vi "ADCP_UI_Update_Receive_List_Table.vi"(8 "error in (no error)":errorcluster, 11 "ADCU_GUI References":T1) -> ()   [LabVIEW 2017]
uses:
  Controls/ADCP_UI/ADCP_UI_Parameters.ctl
  Controls/ADCP_UI/ADCP_UI_Queues.ctl
  Controls/ADCP_UI/ADCP_UI_Continuous_Receiver_States.ctl
  Controls/ADCP_UI/ADCP_Queue_Receive_Log_Queue_Element.ctl
  Controls/Packet/Packet.ctl
  Controls/Packet/Packet_Direction.ctl
  Controls/Packet/Packet_Type.ctl
  Controls/Packet/Packet_Priority.ctl
  Controls/Data Packets/Data_Packet.ctl
  Controls/Data Packets/Parameter.ctl
  Controls/Data Packets/Parameter_Data_Type.ctl
  Controls/Data Packets/Data_Packet_Transmit_Mode.ctl
  <vilib>/Utility/miscctls.llb/LVRowAndColumnTypeDef.ctl
  ADCP_UI_Receive_List_Data_Packets.vi
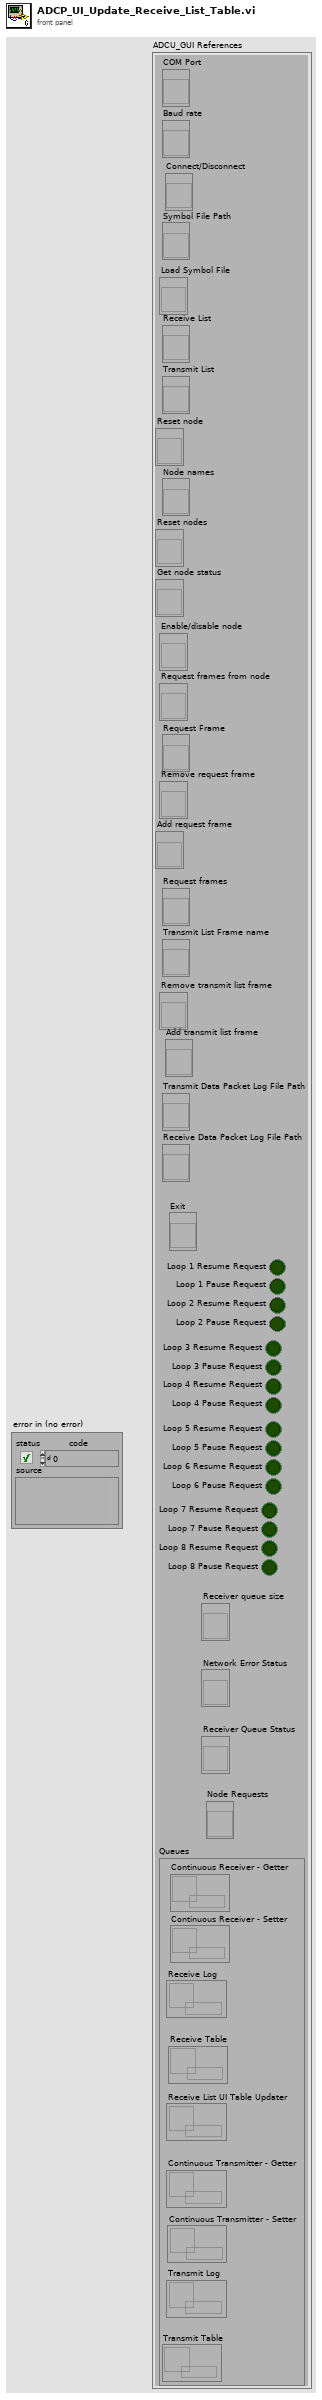
[diagram p1: front panel]
types:
  T1 = typedef "ADCP_UI_Parameters.ctl" = cluster{"COM Port":refnum<vi>, "Baud rate":refnum<vi>, "Symbol File Path":refnum<vi>, "Receive List":refnum<vi>, "Transmit List":refnum<vi>, "Node names":refnum<vi>, "Request Frame":refnum<vi>, "Request frames":refnum<vi>, "Transmit List Frame name":refnum<vi>, "Transmit Data Packet Log File Path":refnum<vi>, "Receive Data Packet Log File Path":refnum<vi>, "Loop 1 Resume Request":bool, "Loop 1 Pause Request":bool, "Loop 2 Resume Request":bool, "Loop 2 Pause Request":bool, "Loop 3 Resume Request":bool, "Loop 3 Pause Request":bool, "Loop 4 Resume Request":bool, "Loop 4 Pause Request":bool, "Loop 5 Resume Request":bool, "Loop 5 Pause Request":bool, "Loop 6 Resume Request":bool, "Loop 6 Pause Request":bool, "Loop 7 Resume Request":bool, "Loop 7 Pause Request":bool, "Loop 8 Resume Request":bool, "Loop 8 Pause Request":bool, "Exit":refnum<vi>, "Connect/Disconnect":refnum<vi>, "Load Symbol File":refnum<vi>, "Reset node":refnum<vi>, "Reset nodes":refnum<vi>, "Get node status":refnum<vi>, "Enable/disable node":refnum<vi>, "Request frames from node":refnum<vi>, "Remove request frame":refnum<vi>, "Add request frame":refnum<vi>, "Remove transmit list frame":refnum<vi>, "Add transmit list frame":refnum<vi>, "Receiver queue size":refnum<vi>, "Network Error Status":refnum<vi>, "Receiver Queue Status":refnum<vi>, "Node Requests":refnum<vi>, "Queues":T2}
  T2 = typedef "ADCP_UI_Queues.ctl" = cluster{"Continuous Receiver - Getter":refnum<queue>, "Continuous Receiver - Setter":refnum<queue>, "Receive Log":refnum<queue>, "Receive Table":refnum<queue>, "Receive List UI Table Updater":refnum<queue>, "Continuous Transmitter - Getter":refnum<queue>, "Continuous Transmitter - Setter":refnum<queue>, "Transmit Log":refnum<queue>, "Transmit Table":refnum<queue>}
  T3 = typedef "Data_Packet.ctl" = cluster{"Packet":T4, "Parameters":T8[], "Last Received Time (ms)":u64, "Receive count":i32, "Transmit count":i32, "Transmit interval (ms)":u32, "Last Transmitted Time (ms)":u64, "Receive interval (ms)":u32, "Transmit_Mode":T10, "Transmit Enable":bool, "Cyclic Transmit interval (ms)":u32}
  T4 = typedef "Packet.ctl" = cluster{"Raw Bytes":u8[], "Checksum":bool, "Direction":T5, "Processed Bytes":u8[], "Node ID":u8, "Packet type":T6, "Frame Data":u32, "Priority":T7, "Frame ID":u8}
  T5 = typedef "Packet_Direction.ctl" = enum16{"Transmit", "Receive", "Bidirectional"}
  T6 = typedef "Packet_Type.ctl" = enum16{"Data", "Connection Management", "Remote Request", "Error/Status"}
  T7 = typedef "Packet_Priority.ctl" = enum16{"LOW", "HIGH"}
  T8 = typedef "Parameter.ctl" = cluster{"Parameter name":string, "Node name":string, "Node ID":u8, "Frame name":string, "Frame ID":u8, "Data type":T9, "Start Bit":i32, "Bit Length":i32, "Factor":dbl, "Offset":dbl, "Minimum":dbl, "Maximum":dbl, "Descriptor":string, "Enum values":string[], "Value":string}
  T9 = typedef "Parameter_Data_Type.ctl" = enum16{"BOOL", "UNSIGNED", "SIGNED", "FLOAT32", "ENUM"}
  T10 = typedef "Data_Packet_Transmit_Mode.ctl" = enum16{"Disabled", "Single", "Cyclic"}
  T11 = typedef "LVRowAndColumnTypeDef.ctl" = cluster{"Row":i32, "Column":i32}
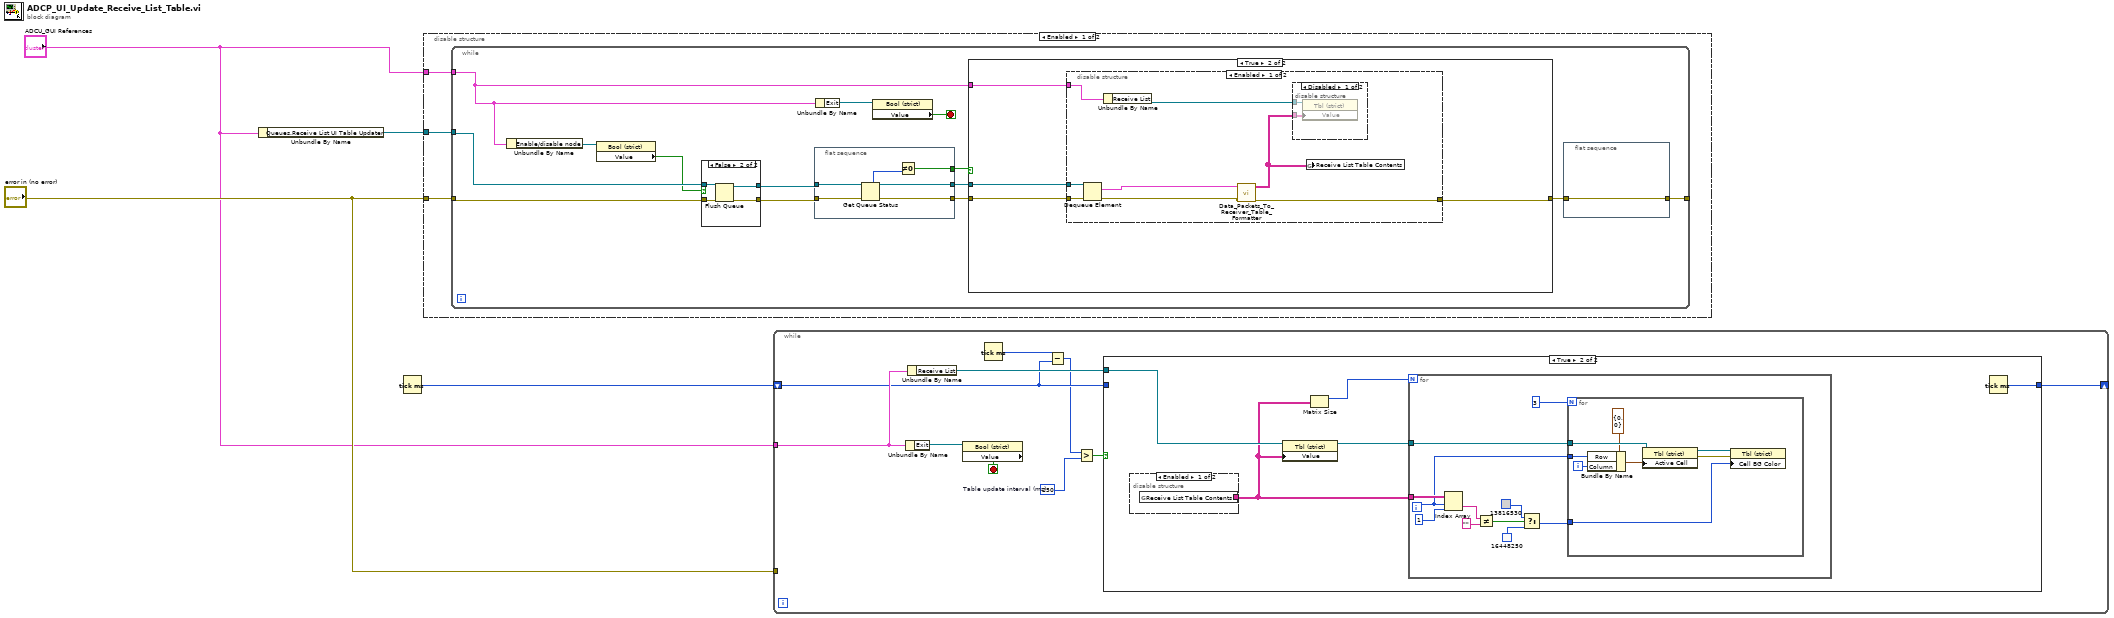
[diagram p0: block diagram]
diagram:
  n1 = Unbundle By Name("ADCU_GUI References") -> ("Queues.Receive List UI Table Updater"=w4:refnum<queue>)
  n2 = Tick Count (ms)() -> (millisecond timer value=w1:u32)
  n3 = disable-structure shown="Enabled" {
    disable-tunnel: "ADCU_GUI References" -> [w7 _]
    disable-tunnel: "error in (no error)" -> [w6 _]
    disable-tunnel: w4 -> [w5 _]
    frame Enabled {
      n4 = while {
        tunnel: w6 -> [w14]
        tunnel: w7 -> [w10]
        tunnel: [w17] -> _
        tunnel: w5 -> [w13]
        stop <- w20 stop-if-true
        n5 = Unbundle By Name(w10) -> ("Enable/disable node"=w9:refnum<vi>)
        n6 = property class="Bool (strict)"(reference=w9) -> ("Value"=w8:bool)  [unwired: 1 in, 2 out]
        n7 = case shown="False" w8 {
          tunnel: w14 -> [w22 w27]
          tunnel: w13 -> [w23 w26]
          tunnel: [w23 w25] -> w12
          tunnel: [w22 w24] -> w11
          frame True {
          }
          frame False {
            n8 = Flush Queue(queue=w26, error in (no error)=w27) -> (queue out=w25:refnum<queue>, error out=w24:errorcluster)  [unwired: 1 out]
          }
        }
        n9 = flat-sequence {
          tunnel: w11 -> [w50]
          tunnel: [w46] -> w19
          tunnel: w12 -> [w49]
          tunnel: [w47] -> w16
          tunnel: [w45] -> w15
          frame #0 {
            n10 = Get Queue Status(queue=w49, error in (no error)=w50) -> (queue out=w45:refnum<queue>, error out=w46:errorcluster, # elements in queue=w48:i32)  [unwired: 1 in, 5 out]
            n11 = Not Equal To 0?(x=w48) -> (x != 0?=w47:bool)
          }
        }
        n12 = Unbundle By Name(w10) -> ("Exit"=w21:refnum<vi>)
        n13 = property class="Bool (strict)"(reference=w21) -> ("Value"=w20:bool)  [unwired: 1 in, 2 out]
        n14 = case shown="True" w16 {
          tunnel: w19 -> [w29 w31]
          tunnel: [w29 w33] -> w18
          tunnel: w10 -> [_ w32]
          tunnel: w15 -> [_ w30]
          frame False {
          }
          frame True {
            n15 = disable-structure shown="Enabled" {
              disable-tunnel: [w41 w44] -> w33
              disable-tunnel: w32 -> [w40 _]
              disable-tunnel: w31 -> [w38 w44]
              disable-tunnel: w30 -> [w36 _]
              frame Enabled {
                n16 = Dequeue Element(queue=w36, error in (no error)=w38) -> (element=w35:T3[], error out=w37:errorcluster)  [unwired: 1 in, 2 out]
                n17 = Unbundle By Name(w40) -> ("Receive List"=w39:refnum<vi>)
                n18 = call "Data_Packets_To_Receiver_Table_Formatter.vi"("error in (no error)"=w37, "Data Packets In"=w35) -> ("error out"=w41:errorcluster, "Table contents"=w34:string[][])  [unwired: 8 in]
                n19 = disable-structure shown="Disabled" {
                  disable-tunnel: w39 -> [w43 _]
                  disable-tunnel: w34 -> [w42 _]
                  frame Disabled {
                    n20 = property class="Tbl (strict)"(reference=w43, "Value"=w42) -> ()  [unwired: 1 in, 2 out]
                  }
                  frame Enabled {
                  }
                }
                n21 = global write "ADCP_UI_Receive_List_Data_Packets.vi" "Receive List Table Contents"(w34) -> ()
              }
              frame Disabled {
              }
            }
          }
        }
        n22 = flat-sequence {
          tunnel: w18 -> [w28]
          tunnel: [w28] -> w17
          frame #0 {
          }
        }
      }
    }
    frame Disabled {
    }
  }
  n23 = while {
    tunnel: "error in (no error)" -> [_]
    tunnel: "ADCU_GUI References" -> [w58]
    shift-right: [w56] -> _
    shift-left: w1 -> [w54]
    stop <- w59 stop-if-true
    w51 = u32 250  # Table update interval (ms)
    n24 = Unbundle By Name(w58) -> ("Exit"=w60:refnum<vi>)
    n25 = Unbundle By Name(w58) -> ("Receive List"=w57:refnum<vi>)
    n26 = property class="Bool (strict)"(reference=w60) -> ("Value"=w59:bool)  [unwired: 1 in, 2 out]
    n27 = Tick Count (ms)() -> (millisecond timer value=w55:u32)
    n28 = Subtract(x=w55, y=w54) -> (x-y=w52:u32)
    n29 = Greater?(x=w52, y=w51) -> (0:w53:bool)
    n30 = case shown="True" w53 {
      tunnel: w57 -> [_ w66]
      tunnel: w54 -> [w61 _]
      tunnel: [w61 w65] -> w56
      frame False {
      }
      frame True {
        n31 = disable-structure shown="Enabled" {
          disable-tunnel: [w86 _] -> w63
          frame Enabled {
            n32 = global read "ADCP_UI_Receive_List_Data_Packets.vi" "Receive List Table Contents"() -> (w86:string[][])
          }
          frame Disabled {
          }
        }
        n33 = property class="Tbl (strict)"(reference=w66, "Value"=w63) -> (reference out=w64:refnum<vi>)  [unwired: 1 in, 1 out]
        n34 = Matrix Size(0:w63) -> (1:w62:i32)  [unwired: 1 out]
        n35 = for {
          N: w62 -> [_]
          tunnel: w64 -> [w73]
          tunnel: w63 -> [w77]
          i -> [w72]
          n36 = Index Array(array=w77, index (row)=w72, index (col)=1 ("disabled index (col)")) -> (element=w75:string)
          n37 = Not Equal?(x=w75, y="") -> (x != y?=w70:bool)
          n38 = Select(t=u32 13816530, s=w70, f=u32 16448250) -> (s? t:f=w67:u32)
          n39 = for {
            N: 3 -> [_]
            tunnel: w73 -> [w85]
            tunnel: w72 -> [w82]
            tunnel: w67 -> [w78]
            i -> [w81]
            n40 = Bundle By Name(cluster=T11 {"Row"=0, "Column"=0} ("Active Cell:Active Cell"), "Row"=w82, "Column"=w81) -> (w83:T11)
            n41 = property class="Tbl (strict)"(reference=w85, "Active Cell"=w83) -> (reference out=w80:refnum<vi>, error out=w79:errorcluster)  [unwired: 1 in]
            n42 = property class="Tbl (strict)"(reference=w80, error in=w79, "Cell BG Color"=w78) -> ()  [unwired: 2 out]
          }
        }
        n43 = Tick Count (ms)() -> (millisecond timer value=w65:u32)
      }
    }
  }
